vi "New State Accessor Dialog.vi"(8 "error in (no error)":errorcluster, 11 "State Accessor Scripter in":refnum<class "State Accessor Scripter.lvclass">) -> (0 "error out":errorcluster, 3 "State Accessor Scripter out":refnum<class "State Accessor Scripter.lvclass">)   [LabVIEW 2015, in "State Accessor Scripter.lvclass"]
uses:
  State Accessor Scripter.lvclass
panel:
  in  "Dynamic/Static":enum32{"Radio Selection 1", "Radio Selection 2"}(radio)
  in  "Type":enum16{"Property", "Accessor"}(ring)
  in  "Access":enum16{"Read", "Write", "Read and Write"}(ring)
  in  "Members":string(tree) caption="State Data members of %s"
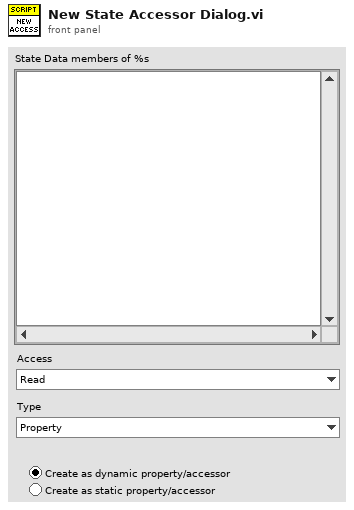
[diagram p1: front panel]
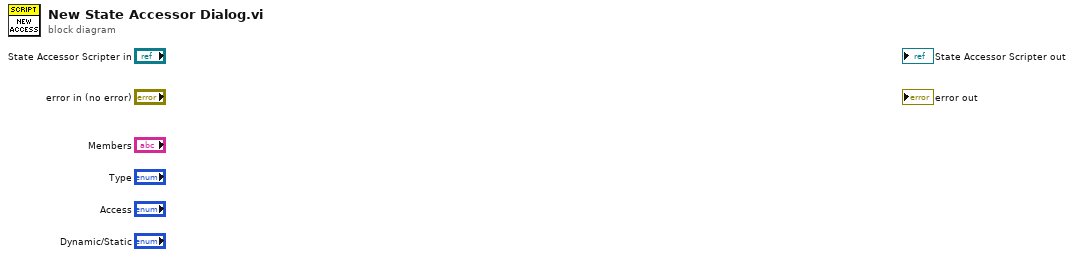
[diagram p0: block diagram]
diagram:
